vi "Sample and Hold.vi"(1 "Hold?":bool, 2 "Input":dbl) -> (0 "Output":dbl)   [LabVIEW 2013]
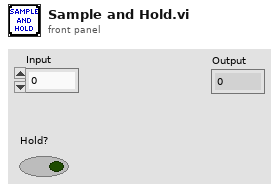
[diagram p1: front panel]
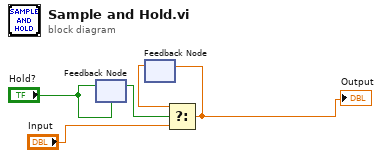
[diagram p0: block diagram]
diagram:
  n1 = feedback #1("Hold?") -> (w1:bool)
  n2 = feedback-in #1("Hold?") -> ()
  n3 = feedback #2() -> (w4:dbl)  [unwired: 1 in]
  n4 = Select(t=w4, s=w1, f="Input") -> (s? t:f=w3:dbl)
  "Output" <- w3
  n5 = feedback-in #2(w3) -> ()
